vi "Stop Core.vi"(10 "final error code":i32, 11 "AMS Gas in":refnum<class "AMS Gas.lvclass">) -> (3 "AMS Gas out":refnum<class "AMS Gas.lvclass">)   [LabVIEW 2015, in "AMS UI.lvlib" / "AMS Gas.lvclass"]
doc: "(<B>Filename</B>: Actor Framework.lvlib:Actor.lvclass:Stop Core.vi)\n\nDefines what the actor does before it stops. Use the <B>final error code</B> input to determine whether the actor shut down in response to an error.\n\nBy default, this method does nothing. A descendant class may override it to define behavior, such as shutting down any processes the actor initiated in its override of the Actor Core method."
uses:
  AMS Gas.lvclass
  AMS Gas.lvclass/AMS Gas.ctl
  <vilib>/ActorFramework/Message Enqueuer/Message Enqueuer.lvclass/Message Enqueuer.ctl
  <vilib>/ActorFramework/Message Enqueuer/Enqueue.vi
  <vilib>/ActorFramework/Message Priority Queue/Priority Enqueue.vi
  <vilib>/ActorFramework/Stop Msg/Stop Msg.lvclass
  <vilib>/ActorFramework/Actor/Actor.lvclass
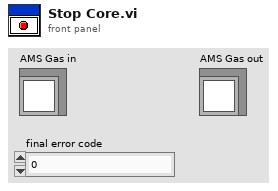
[diagram p1: front panel]
types:
  T1 = cluster{"Log":refnum<class "Message Enqueuer.lvclass">, "Vacuum":refnum<class "Message Enqueuer.lvclass">, "Thermocouples":refnum<class "Message Enqueuer.lvclass">, "Storage":refnum<class "Message Enqueuer.lvclass">, "Samples":refnum<class "Message Enqueuer.lvclass">, "Syringe":refnum<class "Message Enqueuer.lvclass">, "Capillary":refnum<class "Message Enqueuer.lvclass">, "Preparation":refnum<class "Message Enqueuer.lvclass">}
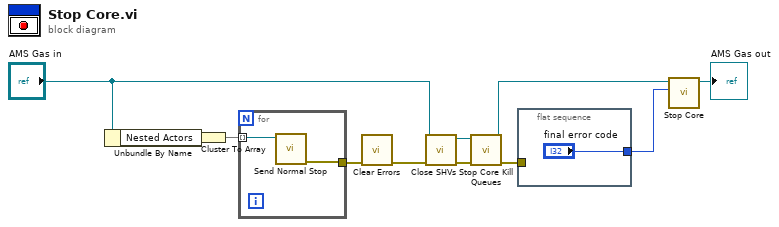
[diagram p0: block diagram]
diagram:
  n1 = Unbundle By Name("AMS Gas in") -> ("Nested Actors"=w9:T1)
  n2 = Cluster To Array(cluster=w9) -> (array=w8:refnum<class "Message Enqueuer.lvclass">[])
  n3 = for {
    tunnel: w8 -> [w13] mode=indexing
    tunnel: [w12] -> w7
    n4 = call <vilib>:"Send Normal Stop.vi"("Message Enqueuer"=w13) -> ("error out"=w12:errorcluster)  [unwired: 10 in]
  }
  n5 = call <vilib>:"Clear Errors.vi"("error in (no error)"=w7) -> ("error out"=w6:errorcluster)  [unwired: 5 in, 1 out]
  n6 = call "Close SHVs.vi"("error in (no error)"=w6, "AMS Gas in"="AMS Gas in") -> ("error out"=w4:errorcluster, "AMS Gas out"=w2:refnum<class "AMS Gas.lvclass">)  [unwired: 8 in]
  n7 = call "Stop Core Kill Queues.vi"("error in (no error)"=w4, "AMS Gas in"=w2) -> ("error out"=w3:errorcluster, "AMS Gas out"=w1:refnum<class "AMS Gas.lvclass">)  [unwired: 8 in]
  n8 = flat-sequence {
    tunnel: ["final error code"] -> w10
    tunnel: w3 -> [_]
    frame #0 {
    }
  }
  n9 = call-parent "Stop Core.vi"("final error code"=w10, "Actor in"=w1) -> ("Actor out"=→"AMS Gas out":refnum<class "AMS Gas.lvclass">)  [unwired: 9 in]
